vi "SRS785_Signal_Analyzer.vi"() -> ()   [LabVIEW 2018]
panel:
  out "time delay":dbl
  out "XY Graph 2":cluster{"Y":dbl[], "Y":dbl[]}[](graph)
  out "token":dbl[](array[numeric])
  out "Elapsed Time (s)":dbl
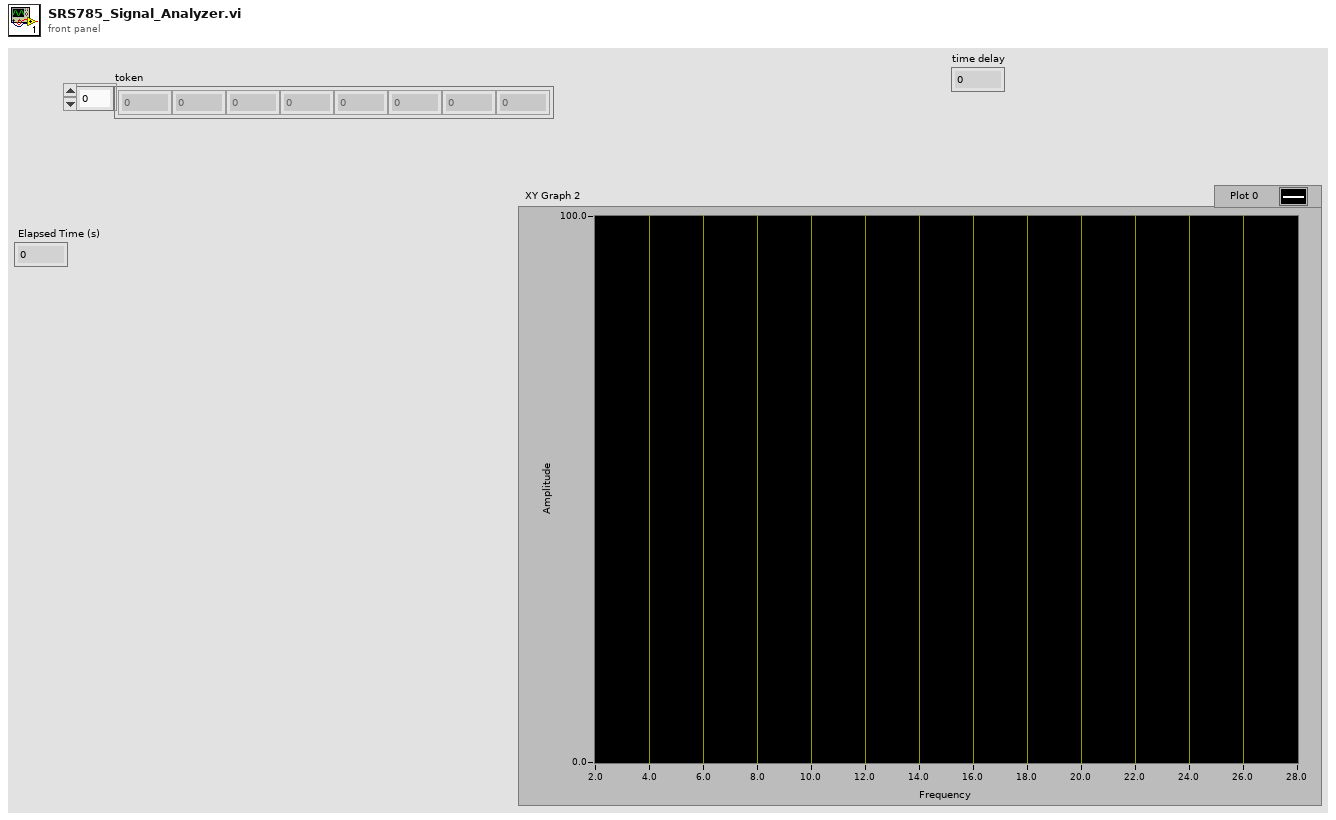
[diagram p1: front panel]
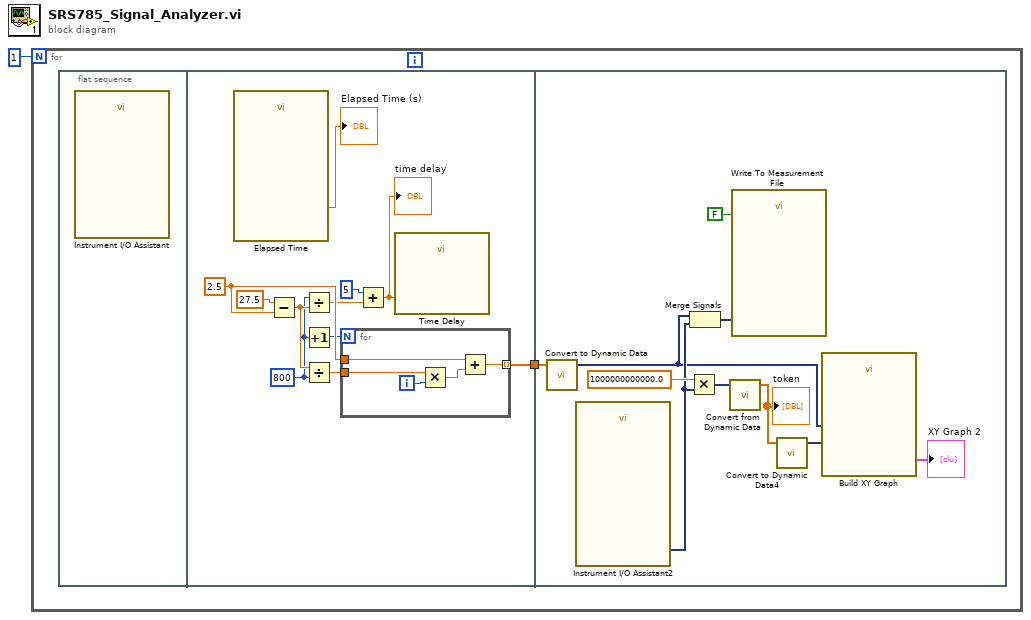
[diagram p0: block diagram]
diagram:
  n1 = for {
    N: 1 -> [_]
    n2 = flat-sequence {
      tunnel: [w5] -> w2
      tunnel: w2 -> [w23]
      frame #0 {
        n3 = call "Instrument I/O Assistant"() -> ()  [unwired: 26 in, 2 out]
      }
      frame #1 {
        w4 = 800
        w11 = 2.5
        n4 = call "Elapsed Time"() -> ("Elapsed Time (s)"=→"Elapsed Time (s)":dbl)  [unwired: 12 in, 7 out]
        n5 = Subtract(x=27.5, y=w11) -> (x-y=w9:dbl)
        n6 = Divide(x=w4, y=w9) -> (x/y=w8:dbl)
        n7 = Increment(x=w4) -> (x+1=w3:i32)
        n8 = Divide(x=w9, y=w4) -> (x/y=w10:dbl)
        n9 = for {
          N: w3 -> [_]
          tunnel: w11 -> [w18]
          tunnel: w10 -> [w16]
          tunnel: [w14] -> w5 mode=indexing
          i -> [w17]
          n10 = Multiply(x=w16, y=w17) -> (x*y=w15:dbl)
          n11 = Add(x=w18, y=w15) -> (x+y=w14:dbl)
        }
        n12 = Add(x=5, y=w8) -> (x+y=w6:dbl)
        "time delay" <- w6
        n13 = call "Time Delay"("Delay Time (s)"=w6) -> ()  [unwired: 10 in, 1 out]
      }
      frame #2 {
        n14 = call "Convert to Dynamic Data"("Array"=w23) -> ("Dynamic Data Type"=w21:dynamicdata)  [unwired: 3 in]
        n15 = call "Instrument I/O Assistant2"() -> ("token"=w22:dynamicdata)  [unwired: 25 in, 2 out]
        n16 = Multiply(x=1000000000000.0, y=w22) -> (x*y=w24:dynamicdata)
        n17 = Merge Signals(w21, w22) -> (w20:dynamicdata)
        n18 = call "Convert from Dynamic Data"("Dynamic Data Type"=w24) -> ("Array"=w27:dbl[])  [unwired: 3 in]
        "token" <- w27
        n19 = call "Write To Measurement File"("Signals"=w20, "Enable"=FALSE) -> ()  [unwired: 15 in, 3 out]
        n20 = call "Convert to Dynamic Data4"("Array"=w27) -> ("Dynamic Data Type"=w26:dynamicdata)  [unwired: 3 in]
        n21 = call "Build XY Graph"("Y Input"=w26, "X Input"=w21) -> ("XY Graph"=→"XY Graph 2":cluster{"X":dbl[], "Y":dbl[]}[])  [unwired: 8 in, 1 out]
      }
    }
  }
